vi "Support_TimerStart.vi"(5 "error in (no error)":errorcluster) -> (13 "Start time":u32, 19 "error out":errorcluster)   [LabVIEW 2009]
doc: "This VI gets the start time in ms."
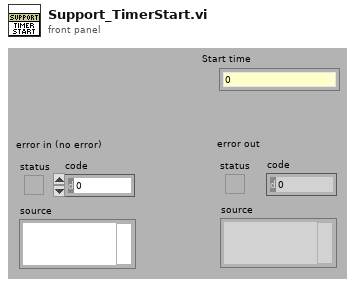
[diagram p1: front panel]
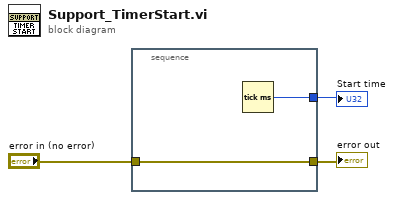
[diagram p0: block diagram]
diagram:
  n1 = stacked-sequence {
    tunnel: [w5] -> w2
    tunnel: "error in (no error)" -> [w5]
    tunnel: [w4] -> w1
    frame #0 {
      n2 = Tick Count (ms)() -> (millisecond timer value=w4:u32)
    }
  }
  "error out" <- w2
  "Start time" <- w1
